vi "Get Debug Data by ID.vi"(8 "error in (no error)":errorcluster, 10 "Message ID":u32, 11 "Debugger in":refnum<class "Debugger.lvclass">) -> (0 "error out":errorcluster, 2 "Debug Data":refnum<class "Debug Data.lvclass">, 3 "Debugger out":refnum<class "Debugger.lvclass">)   [LabVIEW 2020, in "Debugger.lvclass"]
uses:
  Debugger.lvclass
  Debugger.lvclass/Debugger.ctl
  Process/Debug Process.lvclass
  Debug Data/Debug Data.lvclass
  C:/Users/anton/Documents/GitHub/triarc-debugger/source/Process/Debug Process.lvclass
  C:/Users/anton/Documents/GitHub/triarc-debugger/source/Debugger/Debugger.lvclass
  C:/Users/anton/Documents/GitHub/triarc-debugger/source/Debug Data Event/Debug Data Listener.lvclass
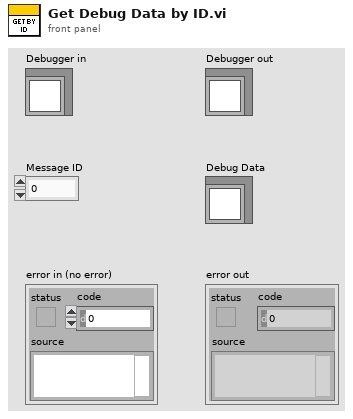
[diagram p1: front panel]
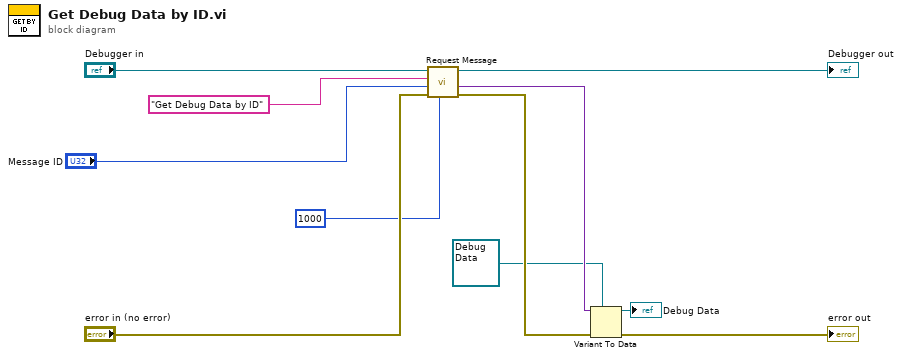
[diagram p0: block diagram]
diagram:
  n1 = call "Request Message.vi"("timeout in ms (-1)"=1000, "error in (no error)"="error in (no error)", "Request Message Data"="Message ID", "Request Message"="Get Debug Data by ID" ("Message"), "Process In"="Debugger in") -> ("error out"=w10:errorcluster, "Response Message Data"=w3:variant, "Process Out"=→"Debugger out":refnum<class "Debugger.lvclass">)  [unwired: 2 in, 2 out]
  n2 = Variant To Data(error in=w10, type=refnum<class "Debug Data.lvclass"> refnum ("Debug Data.lvclass"), Variant=w3) -> (data=→"Debug Data":refnum<class "Debug Data.lvclass">, error out=→"error out":errorcluster)
